vi "SpecObjectArray_get_and_lock_queue.vi"(8 "error in (no error)":errorcluster) -> (0 "error out":errorcluster, 3 "SpecObjects":refnum<class "Spectrometer.lvclass">[](array[class]))   [LabVIEW 2013]
doc: "The VI returns the SpecObject Array. The array is stored in a queue. By dequeueing the array the array becomes locked."
uses:
  Classes/Spectrometer/Spectrometer.lvclass
  global variables.vi
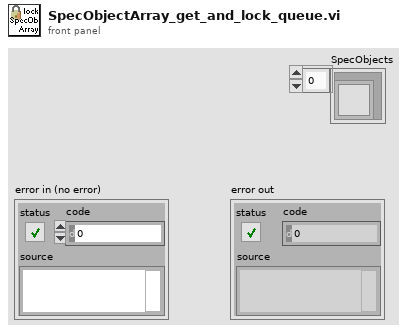
[diagram p1: front panel]
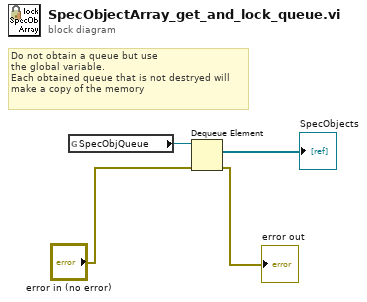
[diagram p0: block diagram]
diagram:
  # "Do not obtain a queue but use\nthe global variable.\nEach obtained queue that is not destryed will\nmake a copy of the memory"
  n1 = global read "global variables.vi" "SpecObjQueue"() -> (w4:refnum<queue>)
  n2 = Dequeue Element(queue=w4, error in (no error)="error in (no error)") -> (element=→"SpecObjects":refnum<class "Spectrometer.lvclass">[], error out=→"error out":errorcluster)  [unwired: 1 in, 2 out]
